vi "SocketWindows.vi"() -> ()   [LabVIEW 2016]
panel:
  in  "stop":bool
  out "Received Message":string
  in  "Porta_Servidor":u16=3535
  in  "IP_Servidor":string="localhost"
  out "ArraySize":i32
  in  "Size Messagem":u32=1500
  out "Sent Mesage":string
  in  "Iterações":i32=1
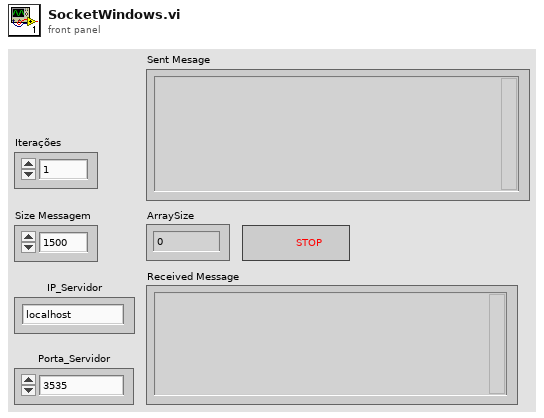
[diagram p1: front panel]
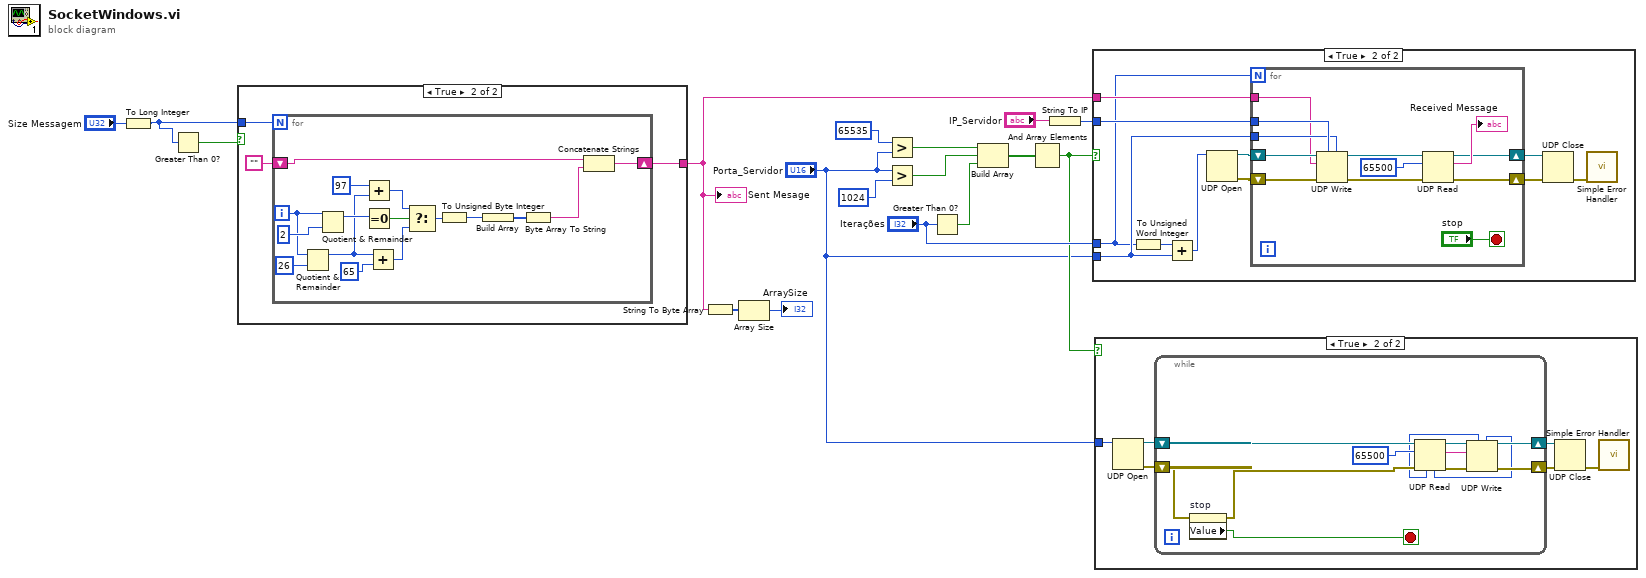
[diagram p0: block diagram]
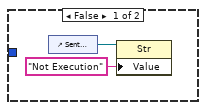
[diagram p2: hidden frame]
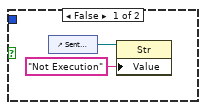
[diagram p3: hidden frame]
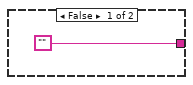
[diagram p4: hidden frame]
diagram:
  n1 = To Long Integer(number="Size Messagem") -> (32bit integer=w16:i32)
  n2 = Greater Than 0?(x=w16) -> (x > 0?=w15:bool)
  n3 = case shown="True" w15 {
    tunnel: w16 -> [_ w20]
    tunnel: ["" w19] -> w3
    frame False {
    }
    frame True {
      n4 = for {
        N: w20 -> [_]
        shift-right: [w26] -> w19
        shift-left: "" -> [w27]
        i -> [w34]
        n5 = Quotient & Remainder(x=w34, y=26) -> (x-y*floor(x/y)=w29:i32)  [unwired: 1 out]
        n6 = Quotient & Remainder(x=w34, y=2) -> (x-y*floor(x/y)=w36:i32)  [unwired: 1 out]
        n7 = Add(x=97, y=w29) -> (x+y=w31:i32)
        n8 = Equal To 0?(x=w36) -> (x = 0?=w35:bool)
        n9 = Add(x=w29, y=65) -> (x+y=w32:i32)
        n10 = Select(t=w31, s=w35, f=w32) -> (s? t:f=w24:i32)
        n11 = To Unsigned Byte Integer(number=w24) -> (unsigned 8bit integer=w23:u8)
        n12 = Build Array(w23) -> (w22:u8[])
        n13 = Byte Array To String(unsigned byte array=w22) -> (string=w25:string)
        n14 = Concatenate Strings(w27, w25) -> (w26:string)
      }
    }
  }
  "Sent Mesage" <- w3
  n15 = String To Byte Array(string=w3) -> (unsigned byte array=w14:u8[])
  n16 = Array Size(array=w14) -> (size(s)=→"ArraySize":i32)
  n17 = Greater?(x=u16 65535, y="Porta_Servidor") -> (0:w9:bool)
  n18 = Greater?(x="Porta_Servidor", y=u16 1024) -> (0:w8:bool)
  n19 = Greater Than 0?(x="Iterações") -> (x > 0?=w7:bool)
  n20 = Build Array(w9, w8, w7) -> (w10:bool[])
  n21 = And Array Elements(Boolean array=w10) -> (logical AND=w2:bool)
  n22 = String To IP(1:"IP_Servidor") -> (0:w5:u32)
  n23 = case shown="True" w2 {
    tunnel: "Porta_Servidor" -> [_ w45]
    tunnel: "Iterações" -> [_ w40]
    tunnel: w5 -> [_ w50]
    tunnel: w3 -> [_ w41]
    frame False {
      n24 = control-ref of="Sent Mesage"() -> (w39:refnum<vi>)
      n25 = property class="Str"(reference=w39, "Value"="Not Execution") -> ()  [unwired: 1 in, 2 out]
    }
    frame True {
      n26 = To Unsigned Word Integer(number=w40) -> (unsigned 16bit integer=w43:u16)
      n27 = Add(x=w43, y=w45) -> (x+y=w44:u16)
      n28 = UDP Open(11:w44) -> (port=w49:refnum<k16>, 0:w48:errorcluster)  [unwired: 4 in, 1 out]
      n29 = for {
        N: w40 -> [_]
        tunnel: w50 -> [w62]
        tunnel: w45 -> [w53]
        tunnel: w41 -> [w52]
        shift-right: [w54] -> w46
        shift-left: w49 -> [w61]
        shift-right: [w55] -> w47
        shift-left: w48 -> [w60]
        stop <- "stop" stop-if-true
        n30 = UDP Write(address=w62, port or service name=w53, connection ID=w61, data in=w52, 8:w60) -> (error out=w59:errorcluster, 3:w58:refnum<k16>)  [unwired: 1 in]
        n31 = UDP Read(connection ID=w58, max size (548)=65500, 8:w59) -> (data out=→"Received Message":string, error out=w55:errorcluster, 3:w54:refnum<k16>)  [unwired: 1 in, 2 out]
      }
      n32 = UDP Close(connection ID=w46, 8:w47) -> (error out=w42:errorcluster)  [unwired: 1 out]
      n33 = call <vilib>:"Simple Error Handler.vi"("error in (no error)"=w42) -> ()  [unwired: 4 in, 5 out]
    }
  }
  n34 = case shown="True" w2 {
    tunnel: "Porta_Servidor" -> [_ w65]
    frame False {
      n35 = control-ref of="Sent Mesage"() -> (w64:refnum<vi>)
      n36 = property class="Str"(reference=w64, "Value"="Not Execution") -> ()  [unwired: 1 in, 2 out]
    }
    frame True {
      n37 = UDP Open(11:w65) -> (port=w70:refnum<k16>, 0:w69:errorcluster)  [unwired: 4 in, 1 out]
      n38 = while {
        shift-right: [w81] -> w67
        shift-left: w70 -> [w82]
        shift-right: [w80] -> w68
        shift-left: w69 -> [w79]
        stop <- w77 stop-if-true
        n39 = property on="stop" class="Bool (strict)"(error in=w79) -> (error out=w78:errorcluster, "Value"=w77:bool)  [unwired: 1 in, 1 out]
        n40 = UDP Read(connection ID=w82, max size (548)=65500, 8:w78) -> (data out=w74:string, error out=w73:errorcluster, 3:w75:refnum<k16>, 4:w72:u16, 6:w71:u32)  [unwired: 1 in]
        n41 = UDP Write(address=w71, port or service name=w72, connection ID=w75, data in=w74, 8:w73) -> (error out=w80:errorcluster, 3:w81:refnum<k16>)  [unwired: 1 in]
      }
      n42 = UDP Close(connection ID=w67, 8:w68) -> (error out=w66:errorcluster)  [unwired: 1 out]
      n43 = call <vilib>:"Simple Error Handler.vi"("error in (no error)"=w66) -> ()  [unwired: 4 in, 5 out]
    }
  }
